vi "ASIC_SET_SUM.vi"(0 "connection ID":refnum<k5>, 1 "Channel Enable":i32(slide) scale=0.0..6.0, 2 "Attenuation Select":i32(slide) scale=0.0..15.0, 3 "Clipping Select":i32(slide)=3 scale=1.0..3.0, 4 "Ib Clip select":i32(slide)=63 scale=0.0..63.0, 5 "error in":errorcluster) -> (14 "connection ID out":refnum<k5>, 19 "error out":errorcluster)   [LabVIEW 2012]
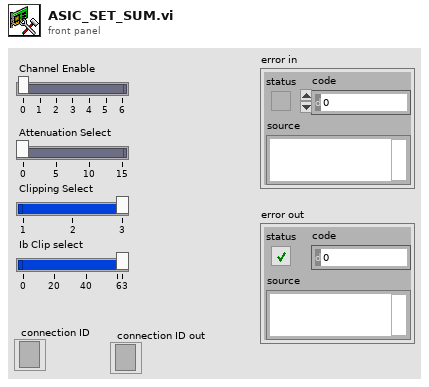
[diagram p1: front panel]
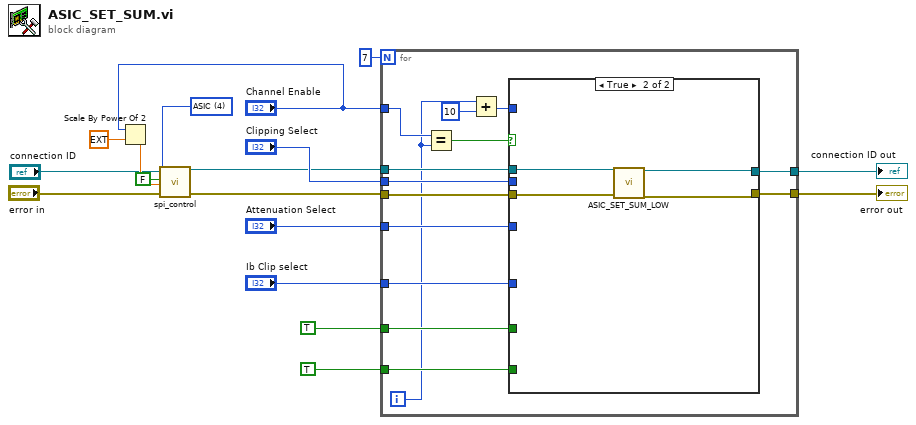
[diagram p0: block diagram]
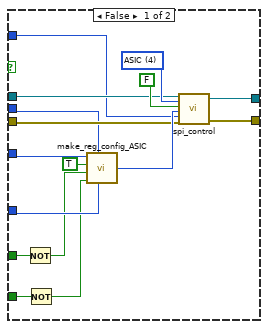
[diagram p2: hidden frame]
diagram:
  w11 = u16 4 items=["Attenuation", "Clipping", "Enable channel", "Delay line", "ASIC"] ("Device")
  n1 = Scale By Power Of 2(n="Channel Enable", x=ext 1.0) -> (x*2^n=w9:ext)
  n2 = call "spi_control.vi"("connection ID"="connection ID", "Device"=w11, "Read/#write"=FALSE, "Data"=w9, "error out 3"="error in") -> ("connection ID out"=w6:refnum<k5>, "error out 2"=w7:errorcluster)  [unwired: 7 in, 6 out]
  n3 = for {
    N: 7 -> [_]
    tunnel: "Clipping Select" -> [w31]
    tunnel: "Ib Clip select" -> [w30]
    tunnel: "Attenuation Select" -> [w29]
    tunnel: w7 -> [w28]
    tunnel: w6 -> [w27]
    tunnel: [w26] -> w2
    tunnel: [w25] -> w1
    tunnel: "Channel Enable" -> [w21]
    tunnel: TRUE ("Clip_en_b") -> [w24]
    tunnel: TRUE ("Att_en_b") -> [w23]
    i -> [w19]
    n4 = Equal?(x=w21, y=w19) -> (x = y?=w22:bool)
    n5 = Add(x=w19, y=10) -> (x+y=w18:i32)
    n6 = case shown="True" w22 {
      tunnel: w31 -> [w38 _]
      tunnel: w30 -> [w41 _]
      tunnel: w29 -> [w40 _]
      tunnel: w28 -> [w39 w51]
      tunnel: w27 -> [w37 w49]
      tunnel: [w35 w50] -> w26
      tunnel: [w36 w48] -> w25
      tunnel: w18 -> [w32 _]
      tunnel: w24 -> [w42 _]
      tunnel: w23 -> [w43 _]
      frame False {
        w46 = u16 4 items=["Attenuation", "Clipping", "Enable channel", "Delay line", "ASIC"] ("Device")
        n7 = Not(x=w42) -> (.not. x?=w34:bool)
        n8 = Not(x=w43) -> (.not. x?=w33:bool)
        n9 = call "make_reg_config_ASIC.vi"("Ib_ClipVb"=w41, "Clip_sel_b"=w38, "Att_en_b"=w33, "Clip_en_b"=w34, "CompBuf_en_b"=TRUE, "Att gain"=w40) -> ("Out reg value"=w44:u32)
        n10 = call "spi_control.vi"("connection ID"=w37, "Device"=w46, "Read/#write"=FALSE, "Data"=w44, "Register or channel"=w32, "error out 3"=w39) -> ("connection ID out"=w36:refnum<k5>, "error out 2"=w35:errorcluster)  [unwired: 6 in, 6 out]
      }
      frame True {
        n11 = call "ASIC_SET_SUM_LOW.vi"("connection ID"=w49, "error in"=w51) -> ("connection ID out"=w48:refnum<k5>, "error out"=w50:errorcluster)  [unwired: 14 in, 2 out]
      }
    }
  }
  "error out" <- w2
  "connection ID out" <- w1
